vi "discarded_open_ab2000.vi"(7 "device type (any)":T1 items=["any"=0, "AB1002"=1002, "AB1004"=1004, "AB1502"=1502, "AB1504"=1504, "AB1902"=1902, "AB1904"=1904, "AB2002"=2002, "AB2004"=2004, "AB2502"=2502, "AB2504"=2504, "AB2902"=2902, "AB2904"=2904], 8 "error in (no error)":errorcluster, 11 "VISA resource name":refnum<visa-resource-name>) -> (0 "error out":errorcluster, 3 "VISA resource name out":refnum<visa-resource-name>)   [LabVIEW 2015, in "Tausand AB1000.lvlib"]
doc: "Sets communication with device.\nWaits 50ms to take into effect the port configuration."
uses:
  <instrlib>/Tausand AB1000/Tausand AB1000.lvlib
  <instrlib>/Tausand AB1000/Public/Controls/deviceTypeRing.ctl
  <vilib>/Instr/_visa.llb/VISA Configure Serial Port (Instr).vi
panel:
  out "IDN out":string
  out "baud rate":u32
  in  "data bits (8)":u16=8
  in  "parity (0:none)":enum16{"None", "Odd", "Even", "Mark", "Space"}(ring)
  in  "flow control (0:none)":u16(ring) items=["None", "XON/XOFF", "RTS/CTS", "XON/XOFF & RTS/CTS", "DTR/DSR", "XON/XOFF & DTR/DSR"]
  in  "stop bits (10: 1 bit)":u16(ring)=10 items=["1.0"=10, "1.5"=15, "2.0"=20]
  # "Discarded VI\nTesting possible changes for future AB2000 devices. DO NOT USE. Saved for future reference only."
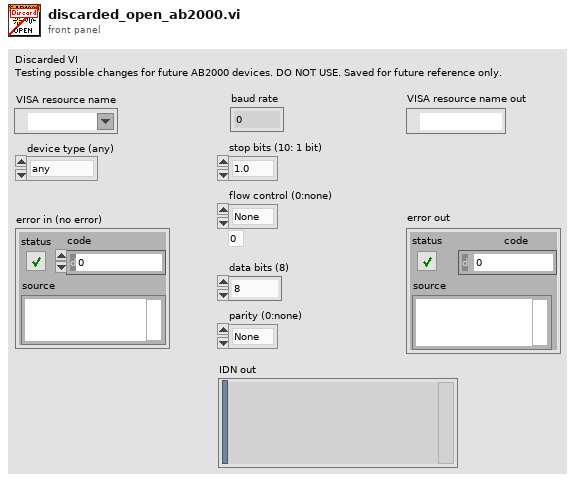
[diagram p1: front panel]
types:
  T1 = typedef "Tausand AB1000.lvlib/deviceTypeRing.ctl" = u16
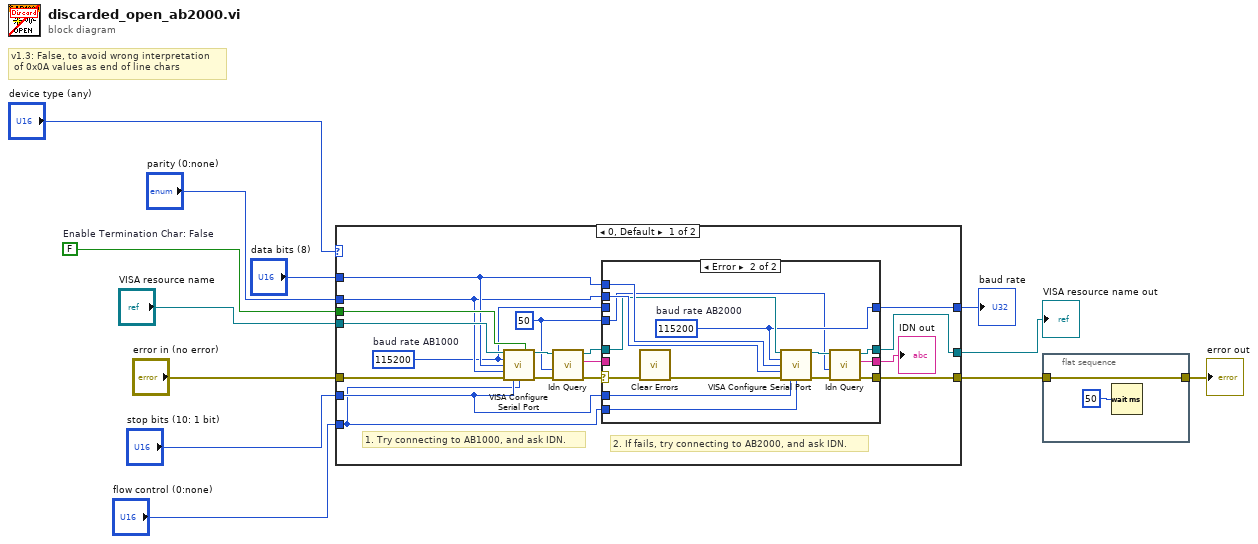
[diagram p0: block diagram]
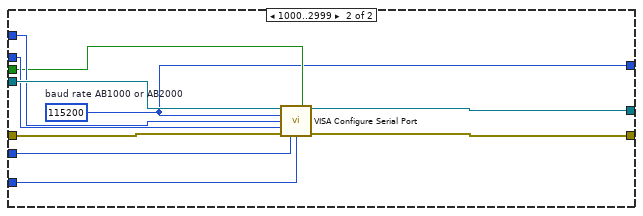
[diagram p3: hidden frame]
diagram:
  w3 = FALSE  # Enable Termination Char: False
  # "v1.3: False, to avoid wrong interpretation\n of 0x0A values as end of line chars"
  n1 = case shown="0, Default" "device type (any)" {
    tunnel: "error in (no error)" -> [w15 w58]
    tunnel: "flow control (0:none)" -> [w23 w57]
    tunnel: "VISA resource name" -> [w30 w56]
    tunnel: "stop bits (10: 1 bit)" -> [w24 w55]
    tunnel: "parity (0:none)" -> [w25 w54]
    tunnel: "data bits (8)" -> [w26 w53]
    tunnel: [w20 w52] -> w6
    tunnel: [w21 w51] -> w4
    tunnel: w3 -> [w29 w50]
    tunnel: [w19 w49] -> w1
    frame 0, Default {
      w17 = u32 50 ("read timeout (1000 ms)")
      w18 = u32 115200  # baud rate AB1000
      # "2. If fails, try connecting to AB2000, and ask IDN."
      # "1. Try connecting to AB1000, and ask IDN."
      n2 = call-poly "VISA Configure Serial Port"("VISA resource name"=w30, "Enable Termination\nChar (T)"=w29, "baud rate (9600)"=w18, "data bits (8)"=w26, "parity (0:none)"=w25, "error in (no error)"=w15, "stop bits (10: 1 bit)"=w24, "flow control (0:none)"=w23) -> ("VISA resource name out"=w27:refnum<visa-resource-name>, "error out"=w28:errorcluster)  [unwired: 6 in]
      n3 = call <instrlib>:"Idn Query.vi"("error in (no error)"=w28, "read timeout (1000 ms)"=w17, "VISA Refnum in"=w27) -> ("error out"=w16:errorcluster, "IDN out"=w13:string, "VISA Refnum out"=w22:refnum<visa-resource-name>)  [unwired: 5 in, 1 out]
      n4 = case shown="Error" w16 {
        selector: w16 -> [w32 w37]
        tunnel: w26 -> [_ w46]
        tunnel: w25 -> [_ w45]
        tunnel: w24 -> [_ w44]
        tunnel: w23 -> [_ w43]
        tunnel: w22 -> [w34 w42]
        tunnel: [w32 w41] -> w21
        tunnel: [w34 w40] -> w20
        tunnel: [w33 w39] -> w19
        tunnel: w18 -> [w33 _]
        tunnel: w17 -> [_ w38]
        tunnel: [w31 w35] -> w14
        tunnel: w13 -> [w31 _]
        frame No Error {
        }
        frame Error {
          w39 = u32 115200  # baud rate AB2000
          n5 = call <vilib>:"Clear Errors.vi"("error in (no error)"=w37) -> ("error out"=w36:errorcluster)  [unwired: 5 in, 1 out]
          n6 = call-poly "VISA Configure Serial Port"("VISA resource name"=w42, "baud rate (9600)"=w39, "data bits (8)"=w46, "parity (0:none)"=w45, "error in (no error)"=w36, "stop bits (10: 1 bit)"=w44, "flow control (0:none)"=w43) -> ("VISA resource name out"=w48:refnum<visa-resource-name>, "error out"=w47:errorcluster)  [unwired: 7 in]
          n7 = call <instrlib>:"Idn Query.vi"("error in (no error)"=w47, "read timeout (1000 ms)"=w38, "VISA Refnum in"=w48) -> ("error out"=w41:errorcluster, "IDN out"=w35:string, "VISA Refnum out"=w40:refnum<visa-resource-name>)  [unwired: 5 in, 1 out]
        }
      }
      "IDN out" <- w14
    }
    frame 1000..2999 {
      w49 = u32 115200  # baud rate AB1000 or AB2000
      n8 = call-poly "VISA Configure Serial Port"("VISA resource name"=w56, "Enable Termination\nChar (T)"=w50, "baud rate (9600)"=w49, "data bits (8)"=w53, "parity (0:none)"=w54, "error in (no error)"=w58, "stop bits (10: 1 bit)"=w55, "flow control (0:none)"=w57) -> ("VISA resource name out"=w52:refnum<visa-resource-name>, "error out"=w51:errorcluster)  [unwired: 6 in]
    }
  }
  "VISA resource name out" <- w6
  "baud rate" <- w1
  n9 = flat-sequence {
    tunnel: [w59] -> w5
    tunnel: w4 -> [w59]
    frame #0 {
      n10 = Wait (ms)(milliseconds to wait=u32 50) -> ()  [unwired: 1 out]
    }
  }
  "error out" <- w5
